vi "Get Name.vi"(8 "error in (no error)":errorcluster, 11 "RFFE RegRead Command in":refnum<class "RFFE RegRead Command.lvclass">) -> (0 "error out":errorcluster, 2 "Name":string, 3 "RFFE RegRead Command out":refnum<class "RFFE RegRead Command.lvclass">)   [LabVIEW 2018, in "MIPI RFFE API.lvlib" / "RFFE RegRead Command.lvclass"]
uses:
  RFFE RegRead Command.lvclass
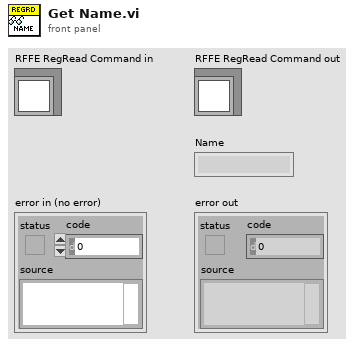
[diagram p1: front panel]
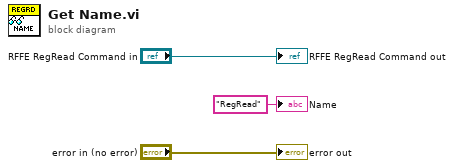
[diagram p0: block diagram]
diagram:
  "error out" <- "error in (no error)"
  "RFFE RegRead Command out" <- "RFFE RegRead Command in"
  "Name" <- "RegRead" ("Name")
